vi "Rohde & Schwarz VNA Read Format.vi"(6 "Channel":i8=1 min=1 max=99 step=1, 7 "Rohde & Schwarz VNA":T1, 8 "error in (no error)":errorcluster, 11 "VISA Resource Name":refnum<visa-resource-name>) -> (0 "error out":errorcluster, 2 "Display Format":T2, 3 "dup VISA Resource Name":refnum<visa-resource-name>)   [LabVIEW 2011]
doc: "This VI for the HP 8753B is used to read the meausurement format.\n\n0 log magnitude\n1 phase\n2 delay\n3 Smith chart\n4 polar\n5 linear magnitude\n6 standing wave ratio\n7 real\n8 imaginary"
uses:
  tests/S Parameter/TypeDefs/SP Measurement Format.ctl
  TypeDefs/Rohde & Schwarz VNA Instrument Info.ctl
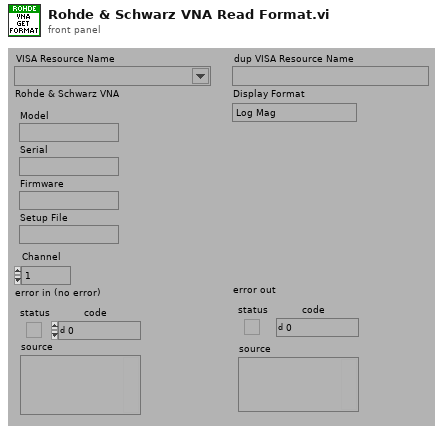
[diagram p1: front panel]
types:
  T1 = typedef "Rohde & Schwarz VNA Instrument Info.ctl" = cluster{"Model":string, "Serial":string, "Firmware":string, "Setup File":string}
  T2 = typedef "SP Measurement Format.ctl" = enum32{"Log Mag", "Phase", "Delay", "Smith (R+jX)", "Polar (Re/Im)", "Linear Mag", "SWR", "Real", "Imaginary", "Smith (Lin/Phase)", "Smith (Log/Phase)", "Smith (Real/Imag)", "Smith (G+jB)", "Polar (Lin/Phase)", "Polar (Log/Phase)", "Expanded Phase", "Positive Phase", "Inverted Smith", "Unwrapped Phase", "Power Out", "Power In", "Linear Mag/Phase", "Log Mag/Phase", "Real/Imaginary"}
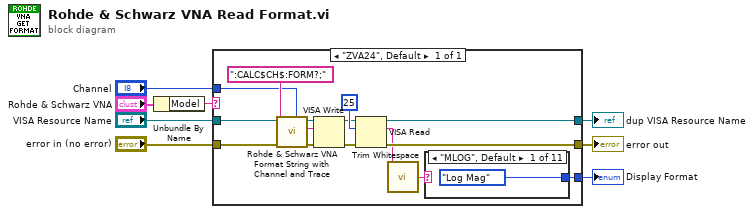
[diagram p0: block diagram]
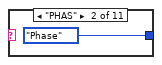
[diagram p2: hidden frame]
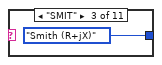
[diagram p3: hidden frame]
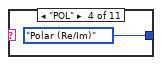
[diagram p4: hidden frame]
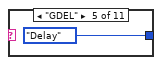
[diagram p5: hidden frame]
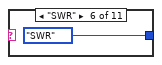
[diagram p6: hidden frame]
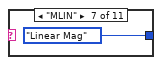
[diagram p7: hidden frame]
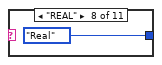
[diagram p8: hidden frame]
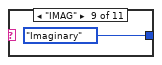
[diagram p9: hidden frame]
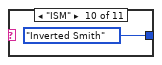
[diagram p10: hidden frame]
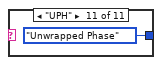
[diagram p11: hidden frame]
diagram:
  n1 = Unbundle By Name("Rohde & Schwarz VNA") -> ("Model"=w2:string)
  n2 = case shown="\"ZVA24\", Default" w2 {
    tunnel: "error in (no error)" -> [w15]
    tunnel: [w18] -> w7
    tunnel: [w10] -> w1
    tunnel: "VISA Resource Name" -> [w16]
    tunnel: [w17] -> w5
    tunnel: "Channel" -> [w9]
    frame "ZVA24", Default {
      n3 = call "Rohde & Schwarz VNA Format String with Channel and Trace.vi"("Trace"=w9, "String"=":CALC$CH$:FORM?;") -> ("String Out"=w13:string)  [unwired: 1 in, 6 out]
      n4 = VISA Write(VISA resource name=w16, write buffer=w13, error in (no error)=w15) -> (VISA resource name out=w20:refnum<visa-resource-name>, error out=w19:errorcluster)  [unwired: 1 out]
      n5 = VISA Read(VISA resource name=w20, byte count=u32 25, error in (no error)=w19) -> (VISA resource name out=w17:refnum<visa-resource-name>, read buffer=w12:string, error out=w18:errorcluster)  [unwired: 1 out]
      n6 = call <vilib>:"Trim Whitespace.vi"("string"=w12) -> ("trimmed string"=w11:string)  [unwired: 1 in]
      n7 = case shown="\"MLOG\", Default" w11 {
        tunnel: [SP_Measurement_Format."Log Mag" ("Display Format") SP_Measurement_Format."Phase" ("Display Format") SP_Measurement_Format."Smith (R+jX)" ("Display Format") SP_Measurement_Format."Polar (Re/Im)" ("Display Format") SP_Measurement_Format."Delay" ("Display Format") SP_Measurement_Format."SWR" ("Display Format") SP_Measurement_Format."Linear Mag" ("Display Format") SP_Measurement_Format."Real" ("Display Format") SP_Measurement_Format."Imaginary" ("Display Format") SP_Measurement_Format."Inverted Smith" ("Display Format") SP_Measurement_Format."Unwrapped Phase" ("Display Format")] -> w10
        frame "MLOG", Default {
        }
        frame "PHAS" {
        }
        frame "SMIT" {
        }
        frame "POL" {
        }
        frame "GDEL" {
        }
        frame "SWR" {
        }
        frame "MLIN" {
        }
        frame "REAL" {
        }
        frame "IMAG" {
        }
        frame "ISM" {
        }
        frame "UPH" {
        }
      }
    }
  }
  "Display Format" <- w1
  "dup VISA Resource Name" <- w5
  "error out" <- w7
